vi "Init.vi"(5 "Bus In":refnum<class "Bus.lvclass">, 7 "Cluster":T1, 8 "error in (no error)":errorcluster, 9 "Init or Array":bool, 10 "Array":dbl[](array[numeric]), 11 "Output in":refnum<class "Output.lvclass">) -> (0 "error out":errorcluster, 2 "Bus Out":refnum<class "Bus.lvclass">, 3 "Output out":refnum<class "Output.lvclass">)   [LabVIEW 2024, in "Output.lvclass"]
uses:
  Output.lvclass
  Scaling/Scaling.lvclass
  Bus/Bus.lvclass
  Output.lvclass/Output.ctl
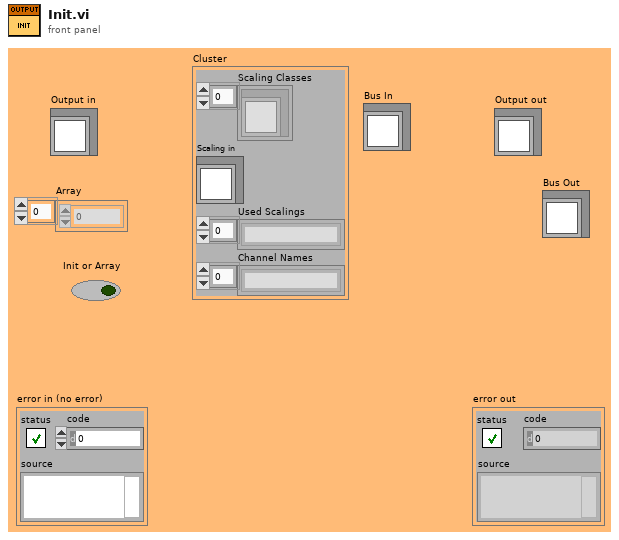
[diagram p1: front panel]
types:
  T1 = cluster{"Scaling Classes":refnum<class "Scaling.lvclass">[], "Scaling in":refnum<class "Scaling.lvclass">, "Used Scalings":string[], "Channel Names":string[]}
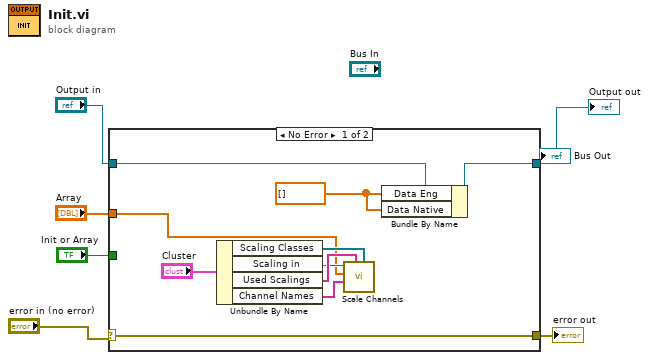
[diagram p0: block diagram]
diagram:
  n1 = case shown="No Error" "error in (no error)" {
    selector: "error in (no error)" -> [w16 w17]
    tunnel: [w16 w17] -> w3
    tunnel: [w15 w18] -> w5
    tunnel: "Output in" -> [w14 w18]
    tunnel: "Init or Array" -> [_ _]
    tunnel: "Array" -> [w7 _]
    frame No Error {
      w13 = dbl[] []
      n2 = Unbundle By Name("Cluster") -> ("Scaling Classes"=w9:refnum<class "Scaling.lvclass">[], "Scaling in"=w10:refnum<class "Scaling.lvclass">, "Used Scalings"=w11:string[], "Channel Names"=w12:string[])
      n3 = call "Scale Channels.vi"("Scaling Classes"=w9, "Used Scalings"=w11, "Channel Names"=w12, "Values In"=w7, "Scaling in"=w10) -> ()  [unwired: 4 in, 3 out]
      n4 = Bundle By Name(cluster=w14, "Data Eng"=w13, "Data Native"=w13) -> (w15:refnum<class "Output.lvclass">)
    }
    frame Error {
    }
  }
  "error out" <- w3
  "Output out" <- w5
